vi "Convert form 2-3 Numbers.vi"(8 "error in (no error)":errorcluster, 9 "data format":bool, 11 "input string":string) -> (0 "error out":errorcluster, 1 "converted numbers":dbl[](array[numeric]) format="%.4e")   [LabVIEW 2018, in "Agilent 87XX Series.lvlib"]
doc: "This VI for the HP8753B is used to convert form 2 and form 3 data arrays. Form 2 is IEEE 32-bit floating point format. Form 3 is IEEE 64-bit floating point format. Both formats are preceded by a 4-byte header which should be included with the \"input string\". As originally written, no VIs in the library use this VI. It is provided as a simple utility should anyone ever need it.\n\n This VI first pulls of the 4 byte header. The second pair of bytes could be converted to a 16-bit number to determine the length of the string which follows. This VI discards the header. \n\n The manuals say that form 2 numbers are 8 bytes and form 3 numbers are 16 bytes. This is because each number is really a pair of numbers. Each number in the pair must be converted separately. This VI is primarily a big loop. Each time through the loop, 4 or 8 bytes are pulled off the string and converted to a number which is then added to an array. Each number is converted with the \"Unflatten from String\" VI or with the \"Type Cast\" VI. For form2 numbers the type converted to should be \"single\"and for form3 numbers the type converted to should be \"double\". The loop executes until there is nothing left in the string."
uses:
  Agilent 87XX Series.lvlib
panel:
  # "form 2\nform 3"
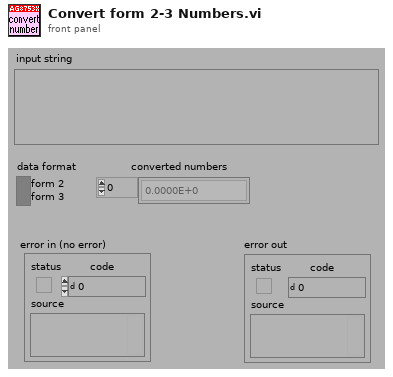
[diagram p1: front panel]
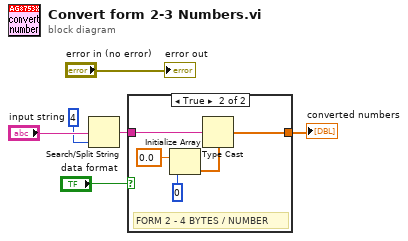
[diagram p0: block diagram]
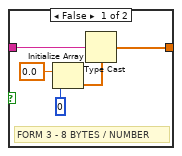
[diagram p2: hidden frame]
diagram:
  n1 = Search/Split String(string="input string", offset (0)=4) -> (match + rest of string=w2:string)  [unwired: 1 in, 2 out]
  n2 = case shown="True" "data format" {
    tunnel: w2 -> [w8 w14]
    tunnel: [w7 w12] -> w1
    frame False {
      # "FORM 3 - 8 BYTES / NUMBER"
      n3 = Initialize Array(0.0, 0) -> (w9:dbl[])
      n4 = Type Cast(type=w9, x=w8) -> (*(type *) &x=w7:dbl[])
    }
    frame True {
      # "FORM 2 - 4 BYTES / NUMBER"
      n5 = Initialize Array(sgl 0.0, 0) -> (w13:sgl[])
      n6 = Type Cast(type=w13, x=w14) -> (*(type *) &x=w12:sgl[])
    }
  }
  "converted numbers" <- w1
  "error out" <- "error in (no error)"
